vi "qSPI.vi"(0 "System no.":i32=1 min=1 max=4 step=1, 5 "error in":errorcluster) -> (14 "Pivot point coordinates":cluster{"R":dbl, "S":dbl, "T":dbl} {"T" format="%.4f"; "S" format="%.4f"; "R" format="%.4f"}, 19 "error out":errorcluster)   [LabVIEW 2020]
doc: "C-886, C-887, F-206- and M-8X0-specific. Returns the pivot point coordinates.\n\nC-887, F-206, M-8X0: Pivot point coordinates (R,S,T) and (X,Y,Z) are valid and identical."
panel:
  # "Hexapod specific. \nReturns the Pivot Point coordinates."
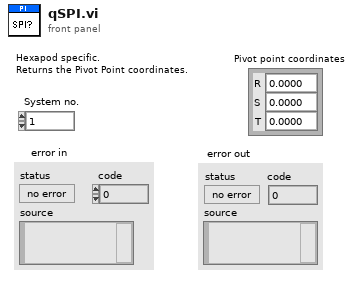
[diagram p1: front panel]
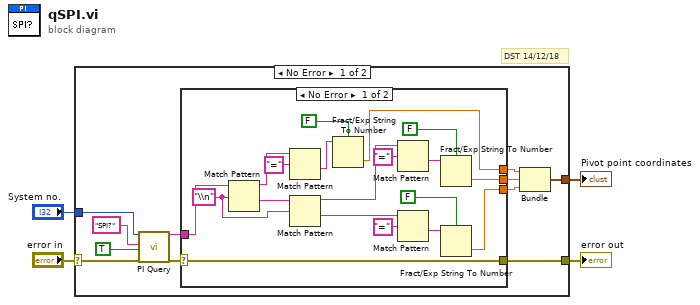
[diagram p0: block diagram]
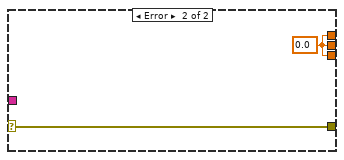
[diagram p2: hidden frame]
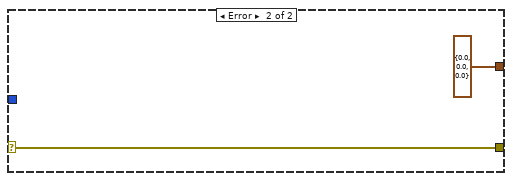
[diagram p3: hidden frame]
diagram:
  # "DST 14/12/18"
  n1 = case shown="No Error" "error in" {
    selector: "error in" -> [w5 w37]
    tunnel: [w14 cluster{dbl, dbl, dbl} {0.0, 0.0, 0.0}] -> w4
    tunnel: "System no." -> [w12 _]
    tunnel: [w6 w37] -> w2
    frame No Error {
      n2 = call "PI Query.vi"("System no."=w12, "String to send"="SPI?", "Attach termination char.?"=TRUE ("Attach Linefeed?"), "error in"=w5) -> ("String read"=w8:string, "error out"=w7:errorcluster)  [unwired: 3 in, 11 out]
      n3 = case shown="No Error" w7 {
        selector: w7 -> [w17 w35]
        tunnel: [w20 w36] -> w11
        tunnel: w8 -> [w21 _]
        tunnel: [w19 w36] -> w10
        tunnel: [w18 w36] -> w9
        tunnel: [w17 w35] -> w6
        frame No Error {
          w16 = "\\n" ("regular expression")
          n4 = Match Pattern(string=w21, regular expression=w16) -> (before substring=w31:string, after substring=w27:string)  [unwired: 3 out]
          n5 = Match Pattern(string=w31, regular expression="=") -> (after substring=w33:string)  [unwired: 4 out]
          n6 = Match Pattern(string=w27, regular expression=w16) -> (before substring=w23:string, after substring=w22:string)  [unwired: 3 out]
          n7 = Fract/Exp String To Number(use system decimal point (T)=FALSE, string=w33) -> (number=w20:dbl)  [unwired: 3 out]
          n8 = Match Pattern(string=w23, regular expression="=") -> (after substring=w29:string)  [unwired: 4 out]
          n9 = Match Pattern(string=w22, regular expression="=") -> (after substring=w25:string)  [unwired: 4 out]
          n10 = Fract/Exp String To Number(use system decimal point (T)=FALSE, string=w29) -> (number=w19:dbl)  [unwired: 3 out]
          n11 = Fract/Exp String To Number(use system decimal point (T)=FALSE, string=w25) -> (number=w18:dbl)  [unwired: 3 out]
        }
        frame Error {
          w36 = 0.0
        }
      }
      n12 = Bundle(w11, w10, w9) -> (w14:cluster{dbl, dbl, dbl})  [unwired: 1 out]
    }
    frame Error {
    }
  }
  "error out" <- w2
  "Pivot point coordinates" <- w4
